vi "读取临时表格数据.vi"(7 "组合框":string(combo), 8 "time 2":string, 9 "表格选择":string(combo)="database1.mdb", 10 "time":string, 11 "table输入":string(combo)) -> (0 "error out":errorcluster, 3 "data":string[][](table))   [LabVIEW 2016]
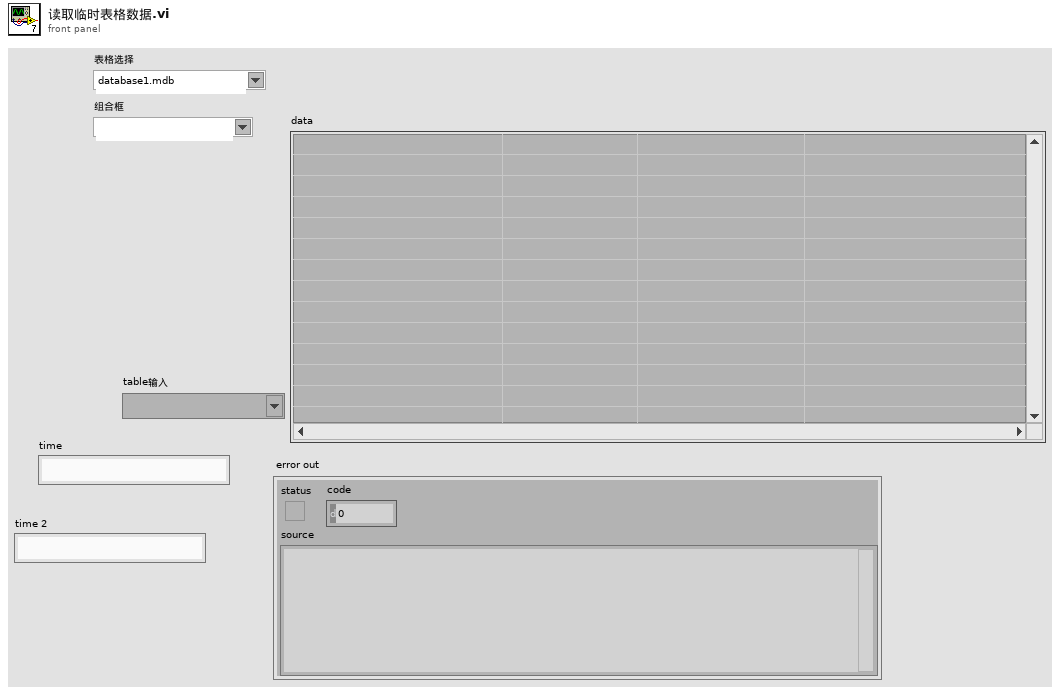
[diagram p1: front panel]
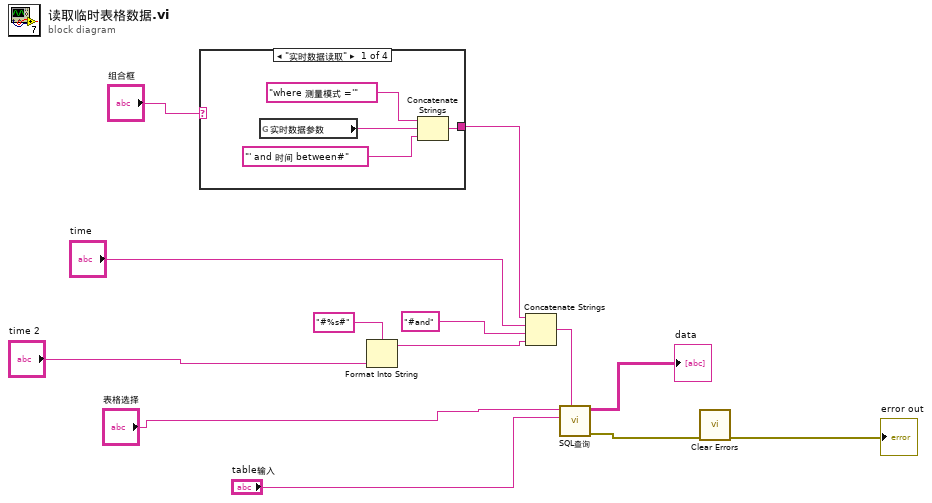
[diagram p0: block diagram]
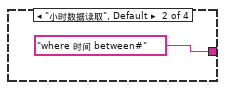
[diagram p2: hidden frame]
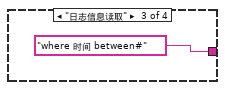
[diagram p3: hidden frame]
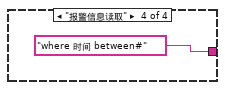
[diagram p4: hidden frame]
diagram:
  n1 = case shown="\"实时数据读取\"" "组合框" {
    tunnel: [w14 "where 时间 between#" ("condition") "where 时间 between#" ("condition") "where 时间 between#" ("condition")] -> w3
    frame "实时数据读取" {
      n2 = global read "全局 实时数据参数.vi" "实时数据参数"() -> (w16:string)
      n3 = Concatenate Strings("where 测量模式 ='" ("condition"), w16, "' and 时间 between#") -> (w14:string)
    }
    frame "小时数据读取", Default {
    }
    frame "日志信息读取" {
    }
    frame "报警信息读取" {
    }
  }
  n4 = Format Into String(format string="#%s#" ("初始字符串"), "time 2") -> (resulting string=w11:string)  [unwired: 2 in, 1 out]
  n5 = Concatenate Strings(w3, "time", "#and" ("字符串"), w11) -> (w13:string)
  n6 = call "SQL查询.vi"("condition"=w13, "table输入"="table输入", "database"="表格选择") -> ("error out"=w8:errorcluster, "data"=→"data":string[][])  [unwired: 7 in]
  n7 = call <vilib>:"Clear Errors.vi"("error in (no error)"=w8) -> ("error out"=→"error out":errorcluster)  [unwired: 5 in, 1 out]
